vi "Set RTDriver VIs File Paths.vi"(8 "error in":errorcluster, 11 "Item Ref in":u64 format="%.0x") -> (0 "error out":errorcluster, 3 "Item Ref out":u64 format="%.0x")   [LabVIEW 2026, in "Template Configuration.lvlib"]
uses:
  Template Configuration.lvlib
  <vilib>/Utility/error.llb/Trim Whitespace (string).vi
  <vilib>/Utility/error.llb/Trim Whitespace One-Sided.vi
  NationalInstruments.VeriStand.SystemStorage
  <vilib>/Utility/LVLibp/NI_PackedLibraryUtility.lvlib
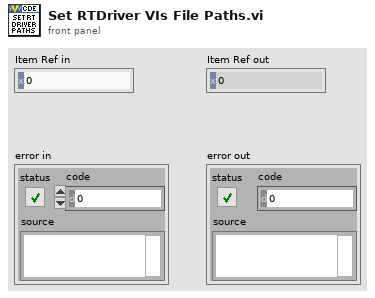
[diagram p1: front panel]
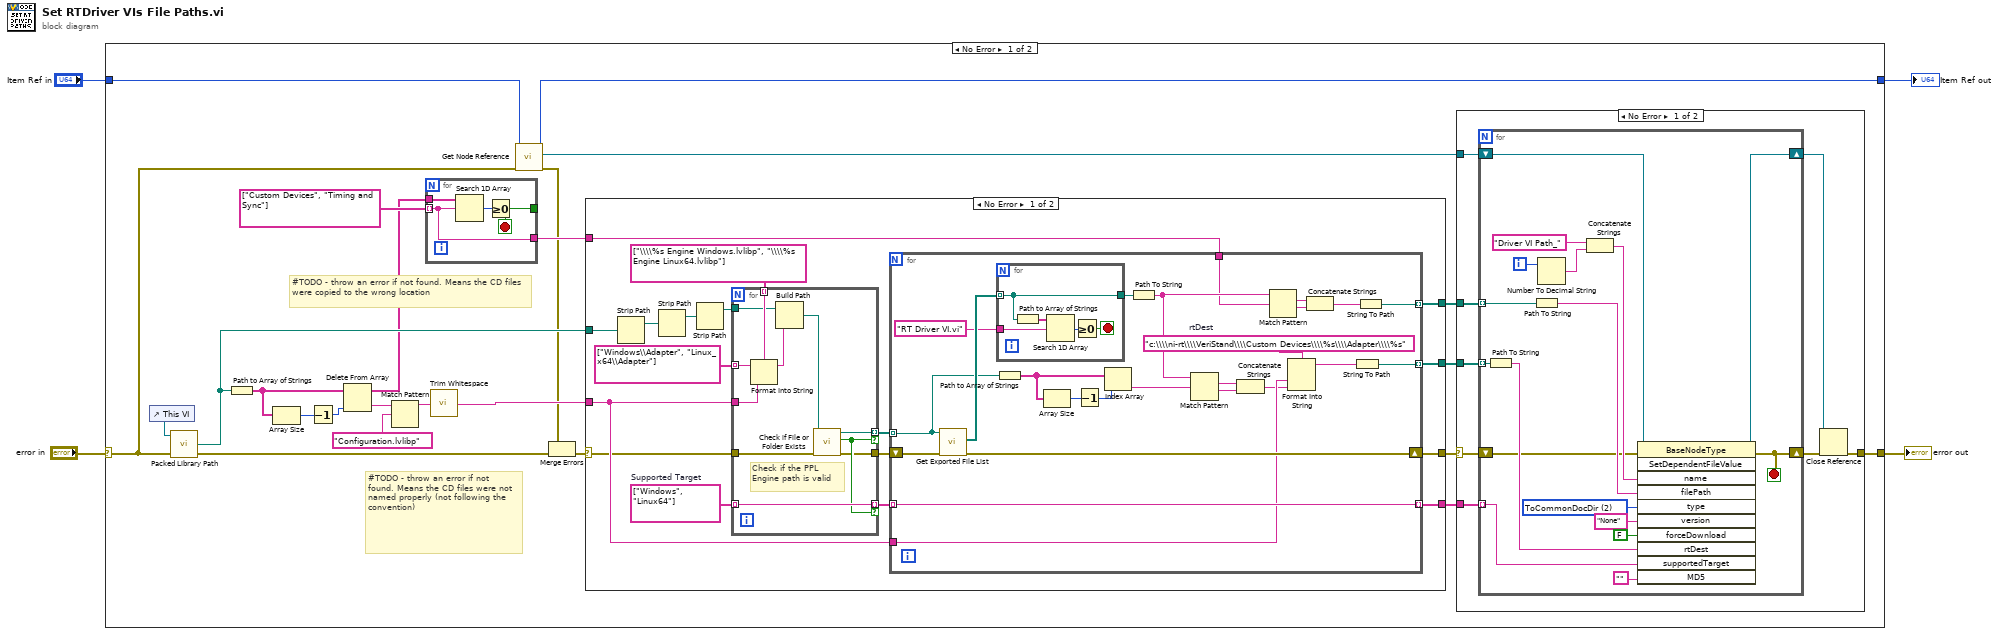
[diagram p0: block diagram]
diagram:
  n1 = case shown="No Error" "error in" {
    selector: "error in" -> [w26 w117]
    tunnel: [w28 w117] -> w4
    tunnel: [w25 w118] -> w3
    tunnel: "Item Ref in" -> [w27 w118]
    frame No Error {
      # "#TODO - throw an error if not found. Means the CD files were not named properly (not following the convention)"
      # "#TODO - throw an error if not found. Means the CD files were copied to the wrong location"
      n2 = control-ref of="This VI"() -> (w24:refnum<vi>)
      n3 = call <vilib>:"Packed Library Path.vi"("error in (no error)"=w26, "vi reference"=w24) -> ("error out"=w7:errorcluster, "packed library path"=w23:path)  [unwired: 1 in, 1 out]
      n4 = Path to Array of Strings(0:w23) -> (2:w22:string[])  [unwired: 1 out]
      n5 = Array Size(array=w22) -> (size(s)=w21:i32)
      n6 = Decrement(x=w21) -> (x-1=w20:i32)
      n7 = Delete From Array(array=w22, index=w20) -> (deleted portion=w19:string, array with subset deleted=w15:string[])  [unwired: 1 in]
      n8 = Match Pattern(string=w19, regular expression="Configuration.lvlibp") -> (before substring=w13:string)  [unwired: 1 in, 3 out]
      n9 = for {
        tunnel: string[] ["Custom Devices", "Timing and Sync"] ("array of strings") -> [w87] mode=indexing
        tunnel: [w89] -> _
        tunnel: w15 -> [w88]
        tunnel: [w87] -> w14
        stop <- w89 stop-if-true
        n10 = Search 1D Array(1D array=w88, element=w87) -> (index of element=w90:i32)  [unwired: 1 in]
        n11 = Greater Or Equal To 0?(x=w90) -> (x >= 0?=w89:bool)
      }
      n12 = call-poly <vilib>:"Trim Whitespace.vi"("string"=w13) -> ("trimmed string"=w17:string)  [unwired: 1 in]
      n13 = call "Get Node Reference.vi"("error in"=w26, "Item Ref in"=w27) -> ("error out"=w6:errorcluster, "Base Node Type"=w5:refnum<k24>, "Item Ref out"=w25:u64)  [unwired: 6 in, 1 out]
      n14 = Merge Errors(w6, w7) -> (w8:errorcluster)
      n15 = case shown="No Error" w8 {
        selector: w8 -> [w35 w86]
        tunnel: w23 -> [w44 _]
        tunnel: [w39 w86] -> w9
        tunnel: w17 -> [w36 _]
        tunnel: w14 -> [w43 _]
        tunnel: [w42 _] -> w12
        tunnel: [w41 _] -> w11
        tunnel: [w40 _] -> w10
        frame No Error {
          w37 = string[] ["Windows", "Linux64"]  # Supported Target
          n16 = Strip Path(path=w44) -> (stripped path=w45:path)  [unwired: 1 out]
          n17 = Strip Path(path=w45) -> (stripped path=w30:path)  [unwired: 1 out]
          n18 = Strip Path(path=w30) -> (stripped path=w29:path)  [unwired: 1 out]
          n19 = for {
            tunnel: string[] ["\\\\%s Engine Windows.lvlibp", "\\\\%s Engine Linux64.lvlibp"] ("Engine Location") -> [w56] mode=indexing
            tunnel: w29 -> [w54]
            tunnel: [w52] -> w32 mode=indexing if=w48
            tunnel: w35 -> [w49]
            tunnel: [w47] -> w34
            tunnel: w37 -> [w51] mode=indexing
            tunnel: [w51] -> w33 mode=indexing if=w48
            tunnel: w36 -> [w50]
            tunnel: string[] ["Windows\\Adapter", "Linux_x64\\Adapter"] ("Engine Location") -> [w46] mode=indexing
            # "Check if the PPL Engine path is valid"
            n20 = Format Into String(format string=w56, initial string=w46, w50) -> (resulting string=w55:string)  [unwired: 1 in, 1 out]
            n21 = Build Path(base path=w54, name or relative path=w55) -> (appended path=w53:path)
            n22 = call <vilib>:"Check if File or Folder Exists.vi"("error in (no error)"=w49, "path"=w53) -> ("error out"=w47:errorcluster, "file or folder exists?"=w48:bool, "dup path"=w52:path)  [unwired: 7 in]
          }
          n23 = for {
            shift-right: [w77] -> w39
            shift-left: w34 -> [w78]
            tunnel: w43 -> [w65]
            tunnel: [w64] -> w42 mode=indexing
            tunnel: [w63] -> w41 mode=indexing
            tunnel: [w62] -> w40 mode=indexing
            tunnel: w36 -> [w60]
            tunnel: w33 -> [w62] mode=indexing
            tunnel: w32 -> [w61] mode=indexing
            w57 = "c:\\\\ni-rt\\\\VeriStand\\\\Custom Devices\\\\%s\\\\Adapter\\\\%s"  # rtDest
            n24 = call <vilib>:"Get Exported File List.vi"("error in (no error)"=w78, "packed library path"=w61) -> ("error out"=w77:errorcluster, "paths"=w80:path[])  [unwired: 7 in, 1 out]
            n25 = Path to Array of Strings(0:w61) -> (2:w68:string[])  [unwired: 1 out]
            n26 = for {
              tunnel: w80 -> [w82] mode=indexing
              tunnel: "RT Driver VI.vi" ("element") -> [w84]
              tunnel: [w82] -> w76
              stop <- w81 stop-if-true
              n27 = Path to Array of Strings(0:w82) -> (2:w85:string[])  [unwired: 1 out]
              n28 = Search 1D Array(1D array=w85, element=w84) -> (index of element=w83:i32)  [unwired: 1 in]
              n29 = Greater Or Equal To 0?(x=w83) -> (x >= 0?=w81:bool)
            }
            n30 = Array Size(array=w68) -> (size(s)=w70:i32)
            n31 = Decrement(x=w70) -> (x-1=w69:i32)
            n32 = Index Array(array=w68, index=w69) -> (element=w67:string)
            n33 = Path To String(path=w76) -> (string=w73:string)
            n34 = Match Pattern(string=w73, regular expression=w67) -> (match substring=w72:string, after substring=w71:string)  [unwired: 1 in, 2 out]
            n35 = Concatenate Strings(w72, w71) -> (w59:string)
            n36 = Match Pattern(string=w73, regular expression=w65) -> (match substring=w75:string, after substring=w74:string)  [unwired: 1 in, 2 out]
            n37 = Format Into String(format string=w57, w60, w59) -> (resulting string=w58:string)  [unwired: 2 in, 1 out]
            n38 = Concatenate Strings(w75, w74) -> (w66:string)
            n39 = String To Path(string=w58) -> (path=w63:path)
            n40 = String To Path(string=w66) -> (path=w64:path)
          }
        }
        frame Error {
        }
      }
      n41 = case shown="No Error" w9 {
        selector: w9 -> [w92 w116]
        tunnel: [w97 w116] -> w28
        tunnel: w12 -> [w96 _]
        tunnel: w11 -> [w95 _]
        tunnel: w10 -> [w94 _]
        tunnel: w5 -> [w93 _]
        frame No Error {
          n42 = for {
            shift-right: [w102] -> w98
            shift-left: w93 -> [w110]
            tunnel: w96 -> [w107] mode=indexing
            tunnel: w95 -> [w106] mode=indexing
            tunnel: w94 -> [w105] mode=indexing
            shift-right: [w99] -> w91
            shift-left: w92 -> [w100]
            i -> [w114]
            stop <- w99 stop-if-true
            w109 = 2 items=["Absolute", "Relative", "ToCommonDocDir", "ToApplicationDataDir"] ("type")
            n43 = Path To String(path=w106) -> (string=w111:string)
            n44 = Path To String(path=w107) -> (string=w112:string)
            n45 = Number To Decimal String(number=w114) -> (decimal integer string=w115:string)  [unwired: 1 in]
            n46 = Concatenate Strings("Driver VI Path_" ("Property name"), w115) -> (w103:string)
            n47 = invoke class="BaseNodeType" method="SetDependentFileValue"(reference=w110, error in=w100, "name"=w103, "filePath"=w112, "type"=w109, "version"="None", "forceDownload"=FALSE, "rtDest"=w111, "supportedTarget"=w105, "MD5"="") -> (reference out=w102:refnum<k24>, error out=w99:errorcluster)  [unwired: 1 in, 9 out]
          }
          n48 = Close Reference(reference=w98, error in (no error)=w91) -> (error out=w97:errorcluster)
        }
        frame Error {
        }
      }
    }
    frame Error {
    }
  }
  "error out" <- w4
  "Item Ref out" <- w3
